vi "PV ActiveLine - Date.vi"(0 "Referenz in":refnum<visa-resource-name>, 1 "W/R":bool, 5 "Day":i8=1 min=1 max=31, 7 "Month":i8=1 min=1 max=12, 9 "Year":i16=2000 min=1970 max=2100, 11 "Fehler (Eingang)":errorcluster) -> (4 "Referenz out":refnum<visa-resource-name>, 6 "outDay":i8=1 min=1 max=31, 8 "outMonth":i8=1 min=1 max=12, 10 "outYear":i16=2000 min=1970 max=2100, 15 "Cluster (Ausgang)":errorcluster)   [LabVIEW 2013, in "PV ActiveLine.lvlib"]
doc: "DAT - Date\n\nTransmit: DAT [,yyyy-mm-dd]\nReceive: yyyy-mm-dd\n\nyyyy-mm-dd = Current date in the format yyyy-mm-dd"
uses:
  <instrlib>/PV ActiveLine/PV ActiveLine.lvlib
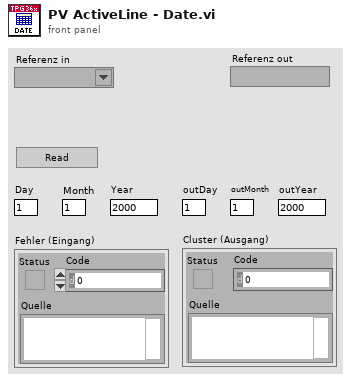
[diagram p1: front panel]
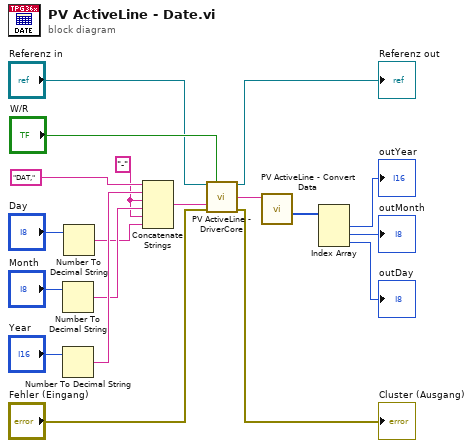
[diagram p0: block diagram]
diagram:
  w9 = "-" ("string")
  n1 = Number To Decimal String(number="Month") -> (decimal integer string=w10:string)  [unwired: 1 in]
  n2 = Number To Decimal String(number="Year") -> (decimal integer string=w11:string)  [unwired: 1 in]
  n3 = Number To Decimal String(number="Day") -> (decimal integer string=w8:string)  [unwired: 1 in]
  n4 = Concatenate Strings("DAT,", w11, w9, w10, w9, w8) -> (w17:string)
  n5 = call <instrlib>:"PV ActiveLine - DriverCore.vi"("Referenz in"="Referenz in", "Write/Read"="W/R", "Command"=w17, "Fehler (Eingang)"="Fehler (Eingang)") -> ("Referenz out"=→"Referenz out":refnum<visa-resource-name>, "String Out"=w5:string, "Cluster (Ausgang)"=→"Cluster (Ausgang)":errorcluster)  [unwired: 9 in]
  n6 = call <instrlib>:"PV ActiveLine - Convert Data.vi"("String in"=w5) -> ("Integer Out"=w4:i32[])  [unwired: 7 in, 3 out]
  n7 = Index Array(array=w4) -> (element #1=→"outYear":i32, element #2=→"outMonth":i32, element #3=→"outDay":i32)  [unwired: 3 in]
